vi "Draw.vi"(8 "error in (no error)":errorcluster, 11 "Rectangle3D in":refnum<class "Rectangle3D.lvclass">) -> (0 "error out":errorcluster, 2 "Picture":picture, 3 "Rectangle3D out":refnum<class "Rectangle3D.lvclass">)   [LabVIEW 2016, in "Rectangle3D.lvclass"]
uses:
  Rectangle3D.lvclass
  C:/Program Files (x86)/National Instruments/LabVIEW 2016/vi.lib/LIEF/Forms/Shape/Shape.lvclass
  <vilib>/LIEF/Forms/Shape/Shape.lvclass/Shape.ctl
  Rectangle3D.lvclass/Rectangle3D.ctl
  <vilib>/LIEF/Forms/Shape/Write Color.vi
  <vilib>/LIEF/Forms/Shape/Read Color.vi
  <vilib>/LIEF/Forms/Rectangle/Rectangle.lvclass
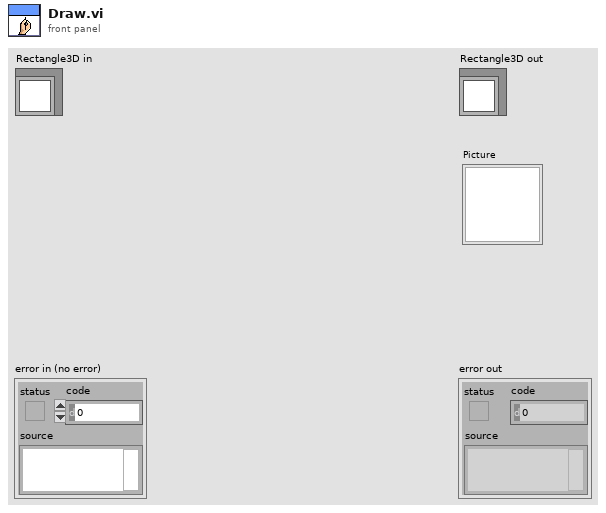
[diagram p1: front panel]
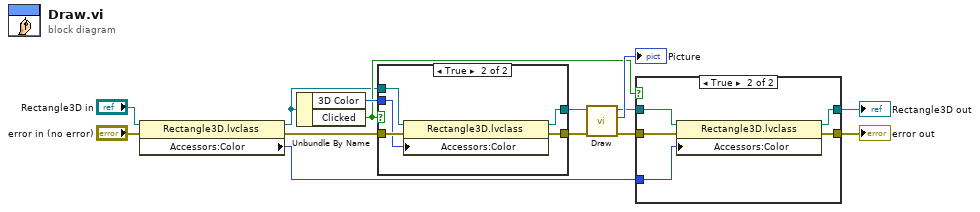
[diagram p0: block diagram]
diagram:
  n1 = property class="Rectangle3D.lvclass"(reference="Rectangle3D in", error in="error in (no error)") -> (reference out=w1:refnum<class "Rectangle3D.lvclass">, error out=w7:errorcluster, "Accessors:Color"=w5:u32)
  n2 = Unbundle By Name(w1) -> ("3D Color"=w13:u32, "Clicked"=w10:bool)
  n3 = case shown="True" w10 {
    tunnel: w1 -> [w16 w21]
    tunnel: w7 -> [w15 w20]
    tunnel: w13 -> [_ w19]
    tunnel: [w16 w18] -> w12
    tunnel: [w15 w17] -> w11
    frame False {
    }
    frame True {
      n4 = property class="Rectangle3D.lvclass"(reference=w21, error in=w20, "Accessors:Color"=w19) -> (reference out=w18:refnum<class "Rectangle3D.lvclass">, error out=w17:errorcluster)
    }
  }
  n5 = call-parent "Draw.vi"("error in (no error)"=w11, "Rectangle in"=w12) -> ("error out"=w3:errorcluster, "Picture"=→"Picture":picture, "Rectangle out"=w6:refnum<class "Rectangle3D.lvclass">)  [unwired: 7 in]
  n6 = case shown="True" w10 {
    tunnel: w6 -> [w23 w28]
    tunnel: w5 -> [_ w27]
    tunnel: [w23 w26] -> w4
    tunnel: w3 -> [w22 w25]
    tunnel: [w22 w24] -> w2
    frame False {
    }
    frame True {
      n7 = property class="Rectangle3D.lvclass"(reference=w28, error in=w25, "Accessors:Color"=w27) -> (reference out=w26:refnum<class "Rectangle3D.lvclass">, error out=w24:errorcluster)
    }
  }
  "error out" <- w2
  "Rectangle3D out" <- w4
